vi "Write Stop Temperature.vi"(8 "error in (no error)":errorcluster, 10 "Stop Temperature":dbl, 11 "SA in":refnum<class "SA.lvclass">) -> (0 "error out":errorcluster, 3 "SA out":refnum<class "SA.lvclass">)   [LabVIEW 2013, in "SA.lvclass"]
uses:
  SA.lvclass
  SA.lvclass/SA.ctl
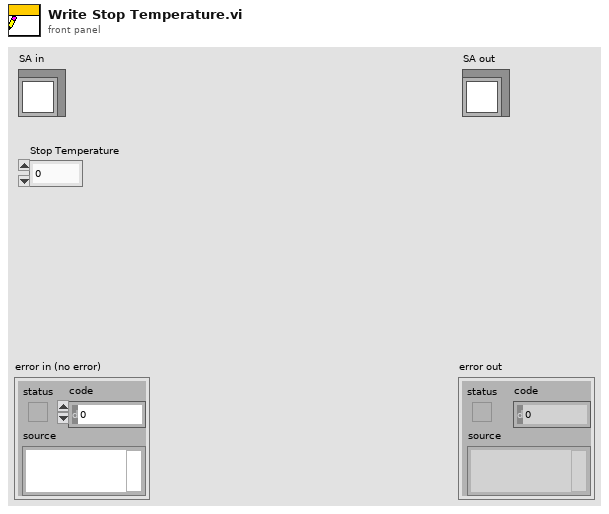
[diagram p1: front panel]
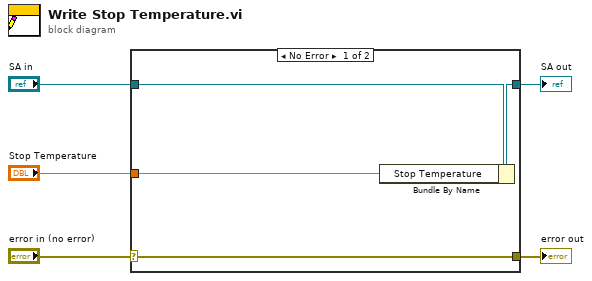
[diagram p0: block diagram]
diagram:
  n1 = case shown="No Error" "error in (no error)" {
    selector: "error in (no error)" -> [w9 w10]
    tunnel: [w9 w10] -> w4
    tunnel: [w7 w11] -> w2
    tunnel: "SA in" -> [w8 w11]
    tunnel: "Stop Temperature" -> [w6 _]
    frame No Error {
      n2 = Bundle By Name(cluster=w8, "Stop Temperature"=w6) -> (w7:refnum<class "SA.lvclass">)
    }
    frame Error {
    }
  }
  "error out" <- w4
  "SA out" <- w2
